vi "write_W.vi"(8 "error in (no error)":errorcluster, 10 "W":dbl[][](array[numeric]), 11 "NMF in":refnum<class "NMF.lvclass">) -> (0 "error out":errorcluster, 3 "NMF out":refnum<class "NMF.lvclass">)   [LabVIEW 2020, in "NMF.lvclass"]
uses:
  NMF.lvclass
  NMF.lvclass/NMF.ctl
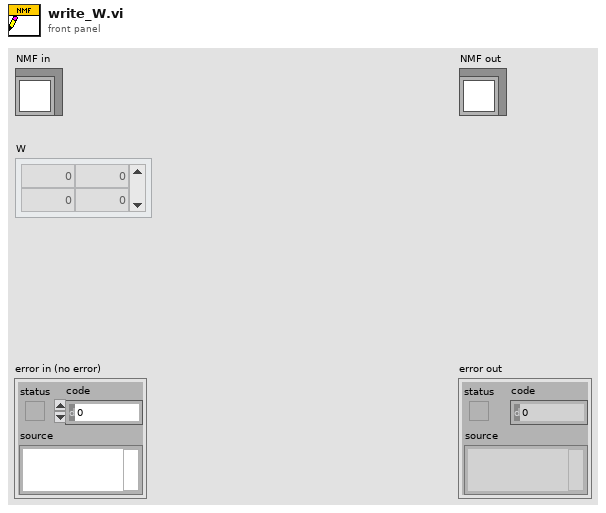
[diagram p1: front panel]
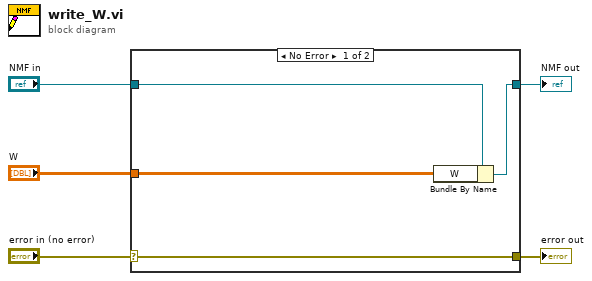
[diagram p0: block diagram]
diagram:
  n1 = case shown="No Error" "error in (no error)" {
    selector: "error in (no error)" -> [w9 w10]
    tunnel: [w9 w10] -> w4
    tunnel: [w7 w11] -> w2
    tunnel: "NMF in" -> [w8 w11]
    tunnel: "W" -> [w6 _]
    frame No Error {
      n2 = Bundle By Name(cluster=w8, "W"=w6) -> (w7:refnum<class "NMF.lvclass">)
    }
    frame Error {
    }
  }
  "error out" <- w4
  "NMF out" <- w2
